vi "Report Gen VI or Documentation.vi"(6 "custom contents options":T14 {"list of controls options"."list which controls?" items=["all controls", "connected controls"]}, 7 "layout options":T2={"orientation (unchanged)"=0, "panel scaling for page (unchanged)"=0, "margins"={"override VI margins (false)"=FALSE, "margins (1.00)"={"top"=1.0, "left"=1.0, "right"=1.0, "bottom"=1.0}, "measurement system (default)"=0}, "printer options"={"destination printer name (current)"="", "printing method (unchanged)"=0, "color or monochrome (unchanged)"=0}, "page header options"={"page headers (unchanged)"=0, "page header content options"={"Include VI Name"=TRUE, "Include VI Path"=TRUE, "Include Last Modification Date"=TRUE, "Include Date Printed"=TRUE, "Include Page Number"=TRUE, "Include VI Icon"=TRUE}}} {"page header options"."page headers (unchanged)" items=["Unchanged", "Include page headers", "Do not include page headers"]; "printer options"."color or monochrome (unchanged)" items=["Unchanged", "Color/grayscale", "Monochrome"]; "printer options"."printing method (unchanged)" items=["Unchanged", "Standard", "PostScript", "Bitmap"]; "panel scaling for page (unchanged)" items=["Unchanged", "No Scaling", "Scale front panel to fit"]; "orientation (unchanged)" items=["Unchanged", "portrait", "landscape"]; "margins"."measurement system (default)" items=["Default", "US", "Metric"]; "margins"."margins (1.00)"."right" format="%.2f"; "margins"."margins (1.00)"."bottom" format="%.2f"; "margins"."margins (1.00)"."top" format="%.2f"; "margins"."margins (1.00)"."left" format="%.2f"}, 8 "error in (no error)":errorcluster, 9 "report type":T1(ring)=enum."HTML", 10 "contents (complete front panel)":T16 items=["Complete front panel", "Visible portion of front panel", "Icon, description, panel and diagram", "Documentation: Using the panel", "Documentation: Using as a subVI", "Documentation: Complete", "Documentation: Custom"], 11 "VI reference":refnum<vi>) -> (0 "error out":errorcluster, 3 "report out":refnum<class "NI_report.lvclass">)   [LabVIEW 2020, in "NI_ReportGenerationCore.lvlib"]
doc: "description"
uses:
  <vilib>/Utility/NIReport.llb/NI_ReportGenerationCore.lvlib
  <vilib>/printing/EasyPrintingControls.llb/contents.ctl
  <vilib>/printing/EasyPrintingControls.llb/custom_contents_options.ctl
  <vilib>/printing/EasyPrintingControls.llb/list_which_controls.ctl
  <vilib>/printing/EasyPrintingControls.llb/layout_options.ctl
  <vilib>/printing/EasyPrintingControls.llb/orientation.ctl
  <vilib>/printing/EasyPrintingControls.llb/panel_scaling_for_page.ctl
  <vilib>/printing/EasyPrintingControls.llb/margins.ctl
  <vilib>/printing/EasyPrintingControls.llb/margin_values.ctl
  <vilib>/printing/EasyPrintingControls.llb/measurement_system.ctl
  <vilib>/printing/EasyPrintingControls.llb/printer_options.ctl
  <vilib>/printing/EasyPrintingControls.llb/printing_method.ctl
  <vilib>/printing/EasyPrintingControls.llb/color_or_monochrome.ctl
  <vilib>/printing/EasyPrintingControls.llb/page_header_options.ctl
  <vilib>/printing/EasyPrintingControls.llb/page_headers.ctl
  <vilib>/printing/EasyPrintingControls.llb/page_header_content_options.ctl
  <vilib>/Utility/NIReport.llb/NI_report.lvclass
  <vilib>/printing/EasyPrintingControls.llb/contents_ENUM.ctl
  <vilib>/printing/ReportDocExtensions.llb/Append Front Panel Image to Report (refnum).vi
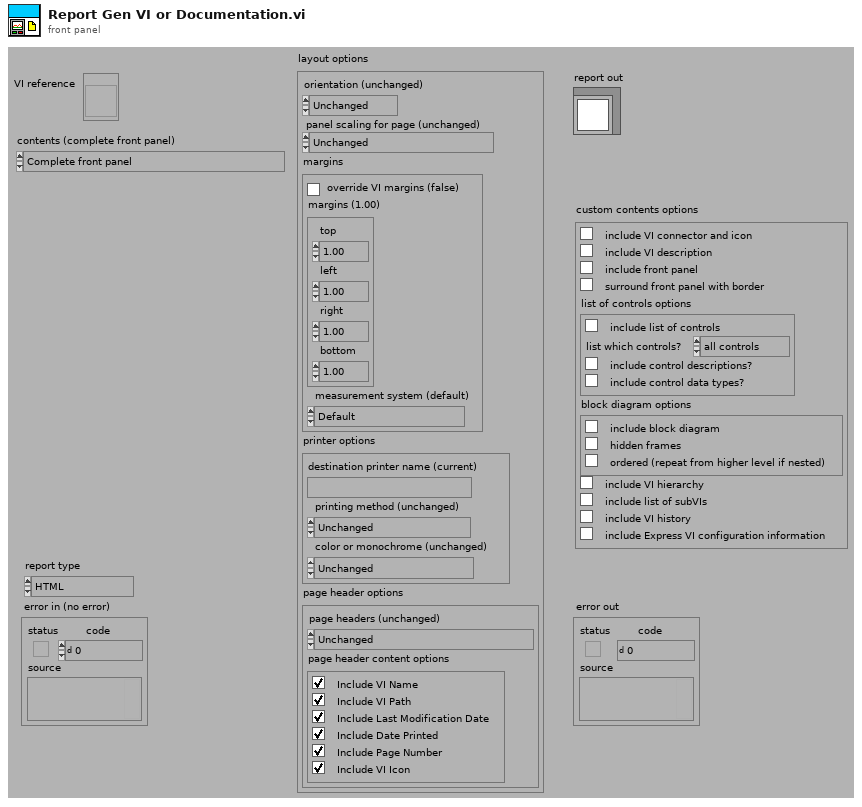
[diagram p1: front panel]
types:
  T1 = enum16{"Standard Report", "HTML", "Word", "Excel"}
  T2 = typedef "NI_ReportGenerationCore.lvlib/layout_options.ctl" = cluster{"orientation (unchanged)":T3, "panel scaling for page (unchanged)":T4, "margins":T5, "printer options":T8, "page header options":T11}
  T3 = typedef "NI_ReportGenerationCore.lvlib/orientation.ctl" = u16
  T4 = typedef "NI_ReportGenerationCore.lvlib/panel_scaling_for_page.ctl" = u16
  T5 = typedef "NI_ReportGenerationCore.lvlib/margins.ctl" = cluster{"override VI margins (false)":bool, "margins (1.00)":T6, "measurement system (default)":T7}
  T6 = typedef "NI_ReportGenerationCore.lvlib/margin_values.ctl" = cluster{"top":dbl, "left":dbl, "right":dbl, "bottom":dbl}
  T7 = typedef "NI_ReportGenerationCore.lvlib/measurement_system.ctl" = u16
  T8 = typedef "NI_ReportGenerationCore.lvlib/printer_options.ctl" = cluster{"destination printer name (current)":string, "printing method (unchanged)":T9, "color or monochrome (unchanged)":T10}
  T9 = typedef "NI_ReportGenerationCore.lvlib/printing_method.ctl" = u16
  T10 = typedef "NI_ReportGenerationCore.lvlib/color_or_monochrome.ctl" = u16
  T11 = typedef "NI_ReportGenerationCore.lvlib/page_header_options.ctl" = cluster{"page headers (unchanged)":T12, "page header content options":T13}
  T12 = typedef "NI_ReportGenerationCore.lvlib/page_headers.ctl" = u16
  T13 = typedef "NI_ReportGenerationCore.lvlib/page_header_content_options.ctl" = cluster{"Include VI Name":bool, "Include VI Path":bool, "Include Last Modification Date":bool, "Include Date Printed":bool, "Include Page Number":bool, "Include VI Icon":bool}
  T14 = typedef "NI_ReportGenerationCore.lvlib/custom_contents_options.ctl" = cluster{"include VI connector and icon":bool, "include VI description":bool, "include front panel":bool, "surround front panel with border":bool, "list of controls options":cluster{"include list of controls":bool, "list which controls?":T15, "include control descriptions?":bool, "include control data types?":bool}, "block diagram options":cluster{"include block diagram":bool, "hidden frames":bool, "ordered (repeat from higher level if nested)":bool}, "include VI hierarchy":bool, "include list of subVIs":bool, "include VI history":bool, "include Express VI configuration information":bool}
  T15 = typedef "NI_ReportGenerationCore.lvlib/list_which_controls.ctl" = u16
  T16 = typedef "NI_ReportGenerationCore.lvlib/contents.ctl" = u16
  T17 = typedef "NI_ReportGenerationCore.lvlib/contents_ENUM.ctl" = enum16{"Complete front panel", "Visible portion of front panel", "Icon, description, panel and diagram", "Documentation: Using the panel", "Documentation: Using as a subVI", "Documentation: Complete", "Documentation: Custom"}
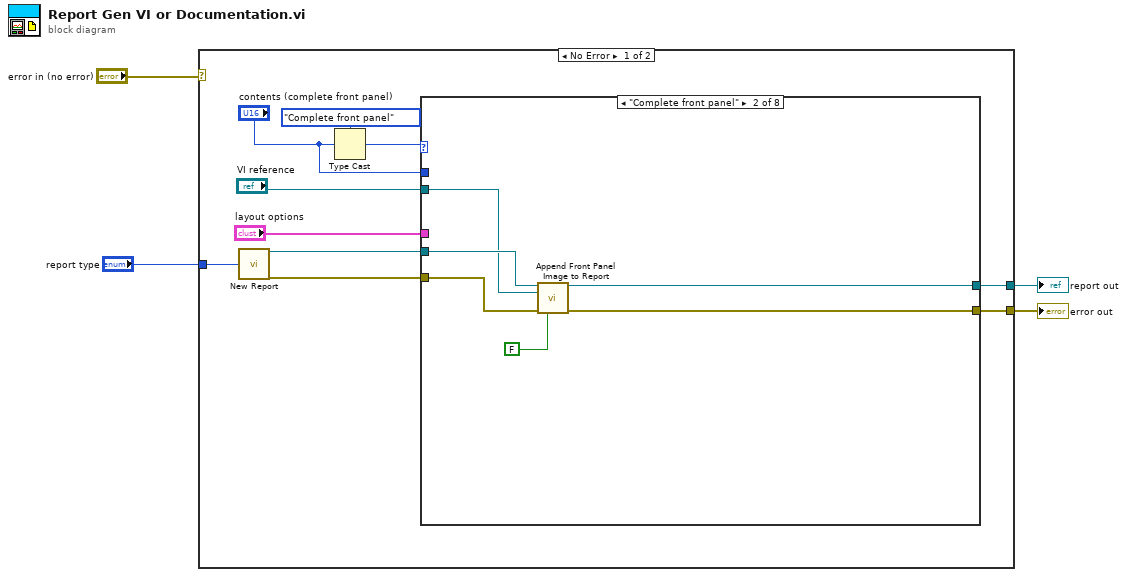
[diagram p0: block diagram]
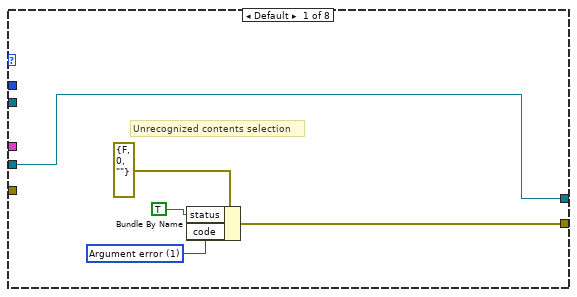
[diagram p2: hidden frame]
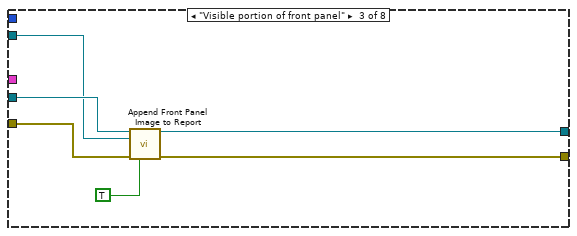
[diagram p3: hidden frame]
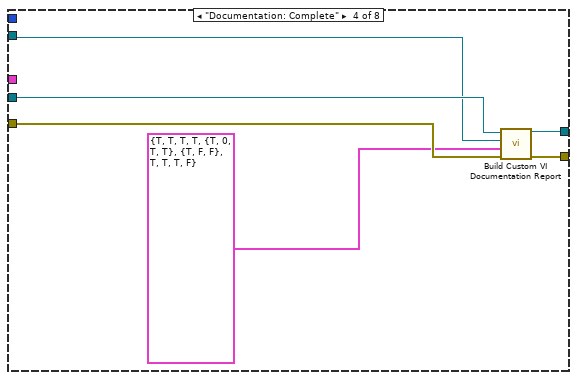
[diagram p4: hidden frame]
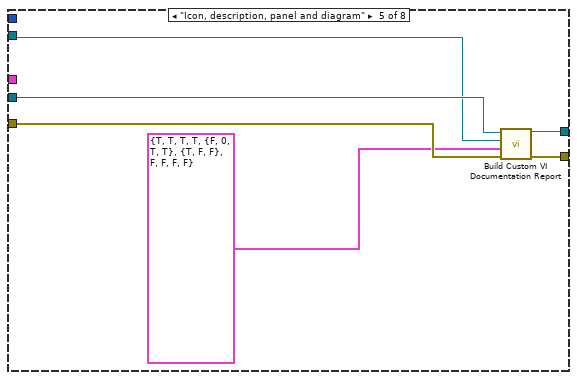
[diagram p5: hidden frame]
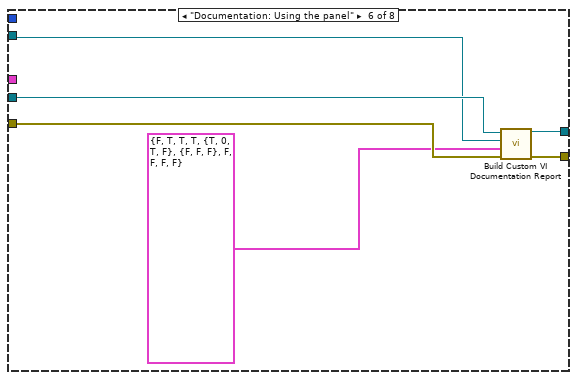
[diagram p6: hidden frame]
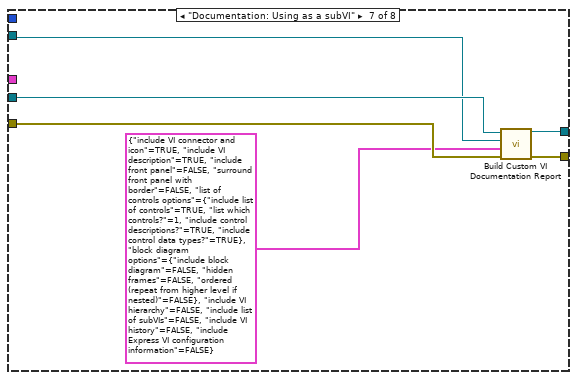
[diagram p7: hidden frame]
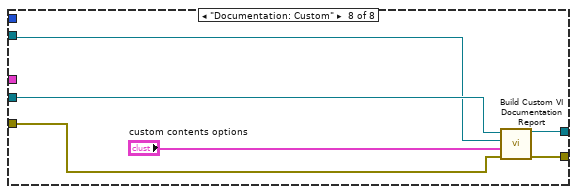
[diagram p8: hidden frame]
diagram:
  n1 = case shown="No Error" "error in (no error)" {
    selector: "error in (no error)" -> [_ w62]
    tunnel: [w7 w62] -> w3
    tunnel: "report type" -> [w11 _]
    tunnel: [w6 _] -> w1
    frame No Error {
      n2 = call <vilib>:"New Report.vi"("report type"=w11) -> ("report out"=w10:refnum<class "NI_report.lvclass">, "error out"=w9:errorcluster)  [unwired: 5 in, 8 out]
      n3 = Type Cast(type=contents_ENUM."Complete front panel" ("Enum"), x="contents (complete front panel)") -> (*(type *) &x=w13:T17)
      n4 = case shown="\"Complete front panel\"" w13 {
        tunnel: "contents (complete front panel)" -> [_ _ _ _ _ _ _ _]
        tunnel: w10 -> [w15 w25 w31 w34 w40 w46 w52 w59]
        tunnel: w9 -> [_ w24 w30 w37 w43 w49 w55 w61]
        tunnel: "VI reference" -> [_ w20 w26 w33 w39 w45 w51 w58]
        tunnel: [w15 w23 w29 w35 w41 w47 w53 w60] -> w6
        tunnel: [w16 w22 w28 w36 w42 w48 w54 w56] -> w7
        tunnel: "layout options" -> [_ _ _ _ _ _ _ _]
        frame Default {
          w18 = 1 items=["No error", "Argument error", "Memory is full", "Out of zone", "End of file", "File already open", "Generic file I/O error", "File not found", "File permission error", "Disk is full", "Duplicate path", "Too many files open", "System feature not enabled", "Resource file not found", "Cannot add resource", "Resource not found", "Image not found", "Image memory error", "Pen does not exist", "Config type invalid", "Config token not found", "Config parse error", "Config memory error", "Bad external code format", "Bad external code offset", "External code not present", "Null window", "Destroy window error", "Null menu", "Print aborted", "Bad print record", "Print driver error", "Windows error during printing", "Memory error during printing", "Print dialog error", "Generic print error", "Invalid device refnum", "Device not found", "Device parameter error", "Device unit error", "Cannot open device", "Device call aborted", "Generic error", "Cancelled by user", "Object ID too low", "Object ID too high", "Object not in heap", "Unknown heap", "Unknown object (invalid DefProc)", "Unknown object (DefProc not in table)", "Message out of range", "Invalid (null) method", "Unknown message", "Manager call not supported", "Bad address", "Network operation in progress", "Network operation timed out", "Connection is busy", "Network attribute not supported", "Network error", "Address in use", "System out of memory", "Connection aborted", "Connection refused", "Not connected", "Already connected", "Connection closed", "Initialization error (interapplication manager)", "Bad occurrence", "Wait on unbound occurrence handler", "Occurrence queue overflow", "Datalog type conflict", "Unused", "Unrecognized type (interapplication manager)", "Memory corrupt", "Failed to make temporary DLL", "Old CIN version", "Drag socket not found", "Failed to load drop-object", "Failed to register OLE object", "Failed to release OLE object", "Format specifier type mismatch", "Unknown format specifier", "Too few format specifiers", "Too many format specifiers", "Scan failed", "Newer CIN version", "Error converting to variant", "Runtime menu error", "Password tampered", "Variant attribute not found", "Incompatible variant data type", "Event data is not available", "Event Store is not present", "Occurrence is not found", "Event Queue is not created", "Event info is not available", "Refnum passed is NULL", "Error retrieving Class GUID", "Error retrieving CoClass GUID", "Error retrieving TypeLib GUID.", "Bad built application magic bytes.", "Specific driver is different from the specific driver associated with the Logical Name.", "There is no session opened to the class driver.", "Max Error", "MAX - Error with config objects", "MAX - Error loading configuration", "MAX - Group not supported"]
          # "Unrecognized contents selection"
          n5 = Bundle By Name(cluster=errorcluster {"status"=FALSE, "code"=0, "source"=""} ("error IO"), "status"=TRUE, "code"=w18) -> (w16:errorcluster)
        }
        frame "Complete front panel" {
          n6 = call-poly <vilib>:"Append Front Panel Image to Report.vi"("report in"=w25, "VI"=w20, "error in (no error)"=w24, "visible area only?"=FALSE ("visible area only")) -> ("report out"=w23:refnum<class "NI_report.lvclass">, "error out"=w22:errorcluster)  [unwired: 4 in, 6 out]
        }
        frame "Visible portion of front panel" {
          n7 = call-poly <vilib>:"Append Front Panel Image to Report.vi"("report in"=w31, "VI"=w26, "error in (no error)"=w30, "visible area only?"=TRUE ("visible area only")) -> ("report out"=w29:refnum<class "NI_report.lvclass">, "error out"=w28:errorcluster)  [unwired: 4 in, 6 out]
        }
        frame "Documentation: Complete" {
          n8 = call <vilib>:"Build Custom VI Documentation Report.vi"("error in (no error)"=w37, "custom contents options"=T14 {"include VI connector and icon"=TRUE, "include VI description"=TRUE, "include front panel"=TRUE, "surround front panel with border"=TRUE, "list of controls options"={"include list of controls"=TRUE, "list which controls?"=0, "include control descriptions?"=TRUE, "include control data types?"=TRUE}, "block diagram options"={"include block diagram"=TRUE, "hidden frames"=FALSE, "ordered (repeat from higher level if nested)"=FALSE}, "include VI hierarchy"=TRUE, "include list of subVIs"=TRUE, "include VI history"=TRUE, "include Express VI configuration information"=FALSE}, "VI reference"=w33, "report in"=w34) -> ("error out"=w36:errorcluster, "report out"=w35:refnum<class "NI_report.lvclass">)  [unwired: 6 out]
        }
        frame "Icon, description, panel and diagram" {
          n9 = call <vilib>:"Build Custom VI Documentation Report.vi"("error in (no error)"=w43, "custom contents options"=T14 {"include VI connector and icon"=TRUE, "include VI description"=TRUE, "include front panel"=TRUE, "surround front panel with border"=TRUE, "list of controls options"={"include list of controls"=FALSE, "list which controls?"=0, "include control descriptions?"=TRUE, "include control data types?"=TRUE}, "block diagram options"={"include block diagram"=TRUE, "hidden frames"=FALSE, "ordered (repeat from higher level if nested)"=FALSE}, "include VI hierarchy"=FALSE, "include list of subVIs"=FALSE, "include VI history"=FALSE, "include Express VI configuration information"=FALSE}, "VI reference"=w39, "report in"=w40) -> ("error out"=w42:errorcluster, "report out"=w41:refnum<class "NI_report.lvclass">)  [unwired: 6 out]
        }
        frame "Documentation: Using the panel" {
          n10 = call <vilib>:"Build Custom VI Documentation Report.vi"("error in (no error)"=w49, "custom contents options"=T14 {"include VI connector and icon"=FALSE, "include VI description"=TRUE, "include front panel"=TRUE, "surround front panel with border"=TRUE, "list of controls options"={"include list of controls"=TRUE, "list which controls?"=0, "include control descriptions?"=TRUE, "include control data types?"=FALSE}, "block diagram options"={"include block diagram"=FALSE, "hidden frames"=FALSE, "ordered (repeat from higher level if nested)"=FALSE}, "include VI hierarchy"=FALSE, "include list of subVIs"=FALSE, "include VI history"=FALSE, "include Express VI configuration information"=FALSE}, "VI reference"=w45, "report in"=w46) -> ("error out"=w48:errorcluster, "report out"=w47:refnum<class "NI_report.lvclass">)  [unwired: 6 out]
        }
        frame "Documentation: Using as a subVI" {
          n11 = call <vilib>:"Build Custom VI Documentation Report.vi"("error in (no error)"=w55, "custom contents options"=T14 {"include VI connector and icon"=TRUE, "include VI description"=TRUE, "include front panel"=FALSE, "surround front panel with border"=FALSE, "list of controls options"={"include list of controls"=TRUE, "list which controls?"=1, "include control descriptions?"=TRUE, "include control data types?"=TRUE}, "block diagram options"={"include block diagram"=FALSE, "hidden frames"=FALSE, "ordered (repeat from higher level if nested)"=FALSE}, "include VI hierarchy"=FALSE, "include list of subVIs"=FALSE, "include VI history"=FALSE, "include Express VI configuration information"=FALSE}, "VI reference"=w51, "report in"=w52) -> ("error out"=w54:errorcluster, "report out"=w53:refnum<class "NI_report.lvclass">)  [unwired: 6 out]
        }
        frame "Documentation: Custom" {
          n12 = call <vilib>:"Build Custom VI Documentation Report.vi"("error in (no error)"=w61, "custom contents options"="custom contents options", "VI reference"=w58, "report in"=w59) -> ("error out"=w56:errorcluster, "report out"=w60:refnum<class "NI_report.lvclass">)  [unwired: 6 out]
        }
      }
    }
    frame Error {
    }
  }
  "error out" <- w3
  "report out" <- w1
